vi "Example Serial Read.vi"(11 "Error IN":errorcluster) -> (15 "Error OUT":errorcluster)   [LabVIEW 2011]
uses:
  <vilib>/rvi/interface/nirviReadWriteControl/nirviReadWriteControl.xnode
  FPGA Bitfiles/JAGM_FPGATarget_FPGAMain_A31A659D.lvbitx
  FPGA Source/FPGA Main.vi
  NiFpgaLv.dll
  <vilib>/Utility/error.llb/Error Cluster From Error Code.vi
  <vilib>/rvi/errors/niLvFpgaAdjustHostInterfaceError.vi
panel:
  out "String":string
  in  "stop":bool
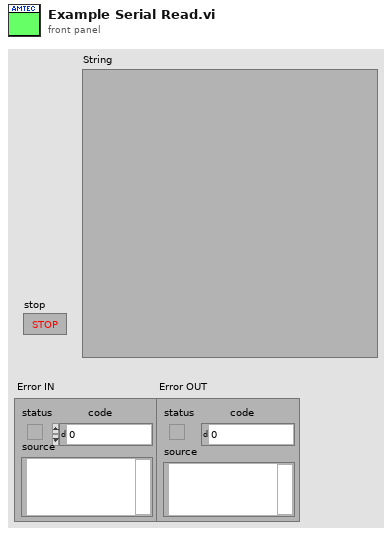
[diagram p1: front panel]
types:
  T1 = cluster{"Data Bit(8)":i32, "Stop Bit":u16, "Baud Rate":u32, "Invert Polarity?":bool, " Mode":bool}[]
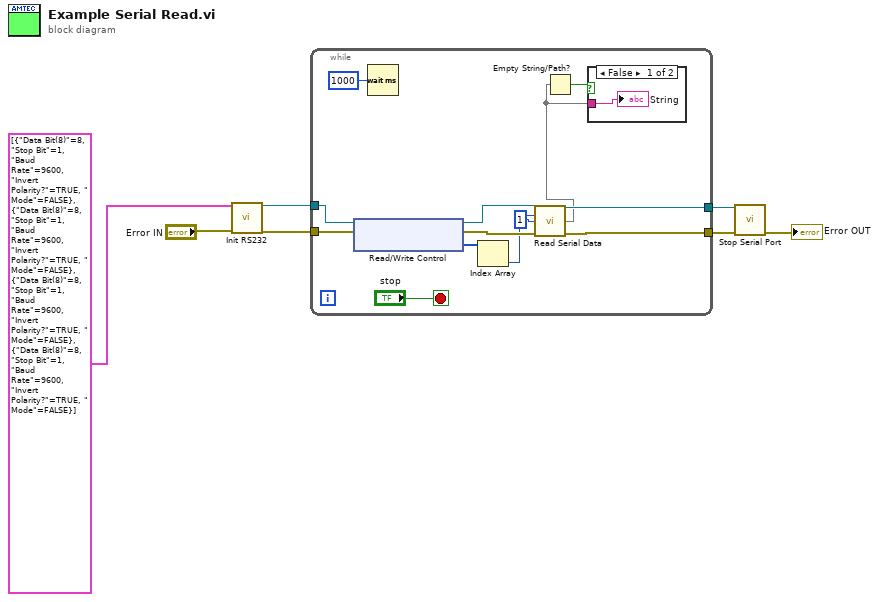
[diagram p0: block diagram]
diagram:
  n1 = call "Init RS232.vi"("Port Settings - 4 Chan"=T1 [{"Data Bit(8)"=8, "Stop Bit"=1, "Baud Rate"=9600, "Invert Polarity?"=TRUE, " Mode"=FALSE}, {"Data Bit(8)"=8, "Stop Bit"=1, "Baud Rate"=9600, "Invert Polarity?"=TRUE, " Mode"=FALSE}, {"Data Bit(8)"=8, "Stop Bit"=1, "Baud Rate"=9600, "Invert Polarity?"=TRUE, " Mode"=FALSE}, {"Data Bit(8)"=8, "Stop Bit"=1, "Baud Rate"=9600, "Invert Polarity?"=TRUE, " Mode"=FALSE}], "error in (no error)"="Error IN") -> ("FPGA Main Reference Out"=w5:refnum<k20>, "error out"=w6:errorcluster)  [unwired: 12 in]
  n2 = while {
    tunnel: w6 -> [w15]
    tunnel: w5 -> [w17]
    tunnel: [w20] -> w4
    tunnel: [w19] -> w3
    stop <- "stop" stop-if-true
    n3 = xnode "Read/Write Control"("FPGA VI Reference In"=w17, "error in"=w15) -> ("FPGA VI Reference Out"=w16:refnum<k20>, "error out"=w14:errorcluster, "Element in Buffer"=w11:u32[])
    n4 = Wait (ms)(milliseconds to wait=u32 1000) -> ()  [unwired: 1 out]
    n5 = Index Array(array=w11) -> (element=w10:u32)  [unwired: 1 in]
    n6 = call "Read Serial Data.vi"("FPGA Main IN"=w16, "Serial Data IN"=w10, 7:1 ("IRQ Number(s)"), "Error IN"=w14) -> ("FPGA VI OUT"=w19:refnum<k20>, 8:w8, "Error OUT"=w20:errorcluster)  [unwired: 8 in, 1 out]
    n7 = Empty String/Path?(string/path=w8) -> (empty?=w12:bool)
    n8 = case shown="False" w12 {
      tunnel: w8 -> [w21 _]
      frame False {
        "String" <- w21
      }
      frame True {
      }
    }
  }
  n9 = call "Stop Serial Port.vi"("FPGA Main Ref"=w3, "Error IN"=w4) -> ("Error OUT"=→"Error OUT":errorcluster)  [unwired: 13 in]
